vi "Map Progress.vi"(6 "Done":bool, 8 "Corner":string, 11 "In":T1) -> (3 "Out":T1)   [LabVIEW 2013]
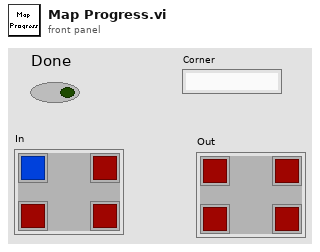
[diagram p1: front panel]
types:
  T1 = cluster{"FL":bool, "FR":bool, "NL":bool, "NR":bool}
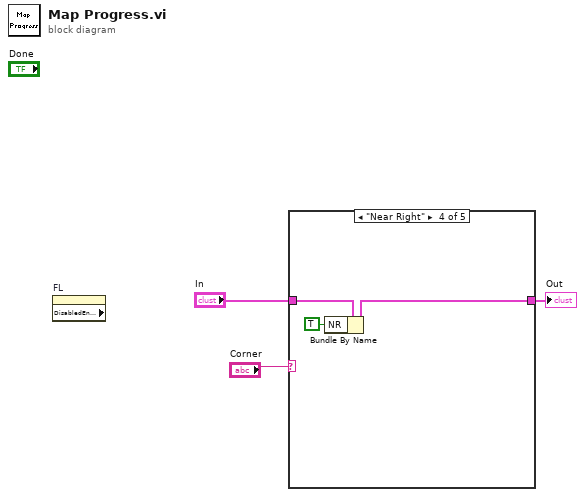
[diagram p0: block diagram]
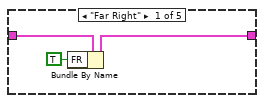
[diagram p2: hidden frame]
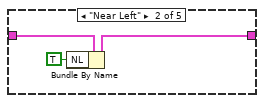
[diagram p3: hidden frame]
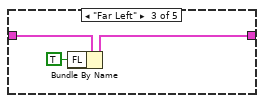
[diagram p4: hidden frame]
diagram:
  n1 = property on="FL" class="Bool (strict)" props=["DisabledEnum"]() -> ()  [unwired: 2 in, 3 out]
  n2 = case shown="\"Near Right\"" "Corner" {
    tunnel: "In" -> [w6 w9 w12 w15 w16]
    tunnel: [w5 w8 w11 w14 w16] -> w1
    frame "Far Right" {
      n3 = Bundle By Name(cluster=w6, "FR"=TRUE ("1")) -> (w5:T1)
    }
    frame "Near Left" {
      n4 = Bundle By Name(cluster=w9, "NL"=TRUE ("1")) -> (w8:T1)
    }
    frame "Far Left" {
      n5 = Bundle By Name(cluster=w12, "FL"=TRUE ("1")) -> (w11:T1)
    }
    frame "Near Right" {
      n6 = Bundle By Name(cluster=w15, "NR"=TRUE ("1")) -> (w14:T1)
    }
    frame Default {
    }
  }
  "Out" <- w1
